vi "Main.vi"() -> (0 "error out":errorcluster)   [LabVIEW 2010, in "Sound Demo.lvclass"]
doc: "This is the top-level VI that starts the Sound Player Demo application."
uses:
  Sound Demo.lvclass
  Application/Application.lvclass
panel:
  # "This is the top-level VI of the \nSound Player Demo project."
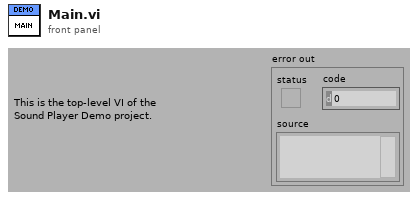
[diagram p1: front panel]
types:
  T1 = enum32{"invalid app kind", "Development System", "Run Time System", "Student Edition", "Embedded LabVIEW", "Evaluation", "Custom"}
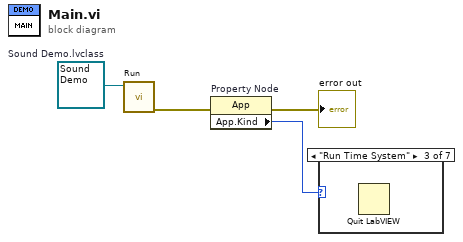
[diagram p0: block diagram]
diagram:
  w4 = refnum<class "Sound Demo.lvclass"> refnum  # Sound Demo.lvclass
  n1 = call "Run.vi"("Application in"=w4) -> ("error out"=w3:errorcluster)  [unwired: 9 in, 1 out]
  n2 = property on="Property Node" class="App"(error in=w3) -> (error out=→"error out":errorcluster, "App.Kind"=w1:T1)  [unwired: 1 in, 1 out]
  n3 = case shown="\"Run Time System\"" w1 {
    frame "invalid app kind", Default {
    }
    frame "Development System" {
    }
    frame "Run Time System" {
      n4 = Quit LabVIEW() -> ()  [unwired: 1 in]
    }
    frame "Student Edition" {
    }
    frame "Embedded LabVIEW" {
    }
    frame "Evaluation" {
    }
    frame "Custom" {
    }
  }
